vi "ejerciciofig5-Martin.vi"() -> ()   [LabVIEW 2020]
panel:
  in  "Fila":dbl[](array[numeric])
  in  "Index fila":i32
  in  "Seleccion":u8
  out "Salida":dbl[][](array[numeric])
  in  "Entrada":dbl[][](array[numeric])
  # "Digite solamente 1 o 2, segun requiera"
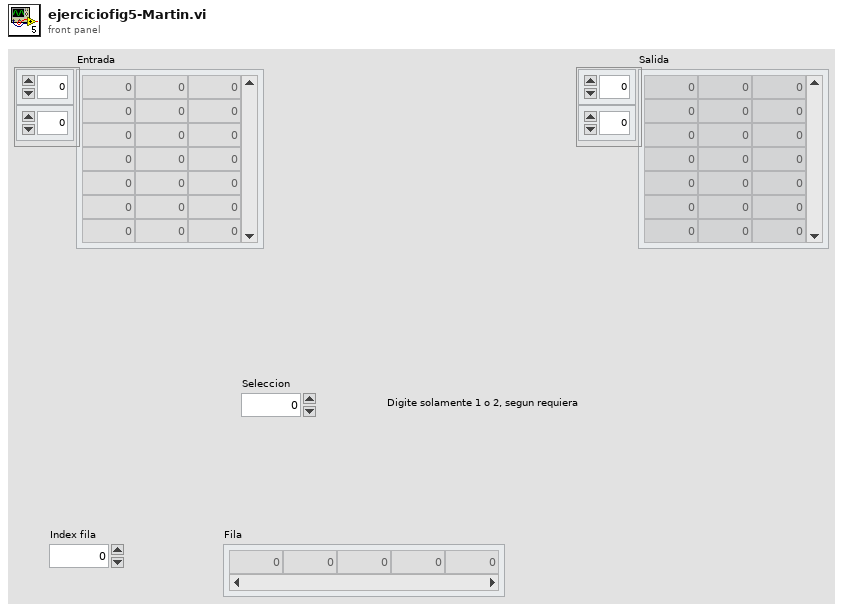
[diagram p1: front panel]
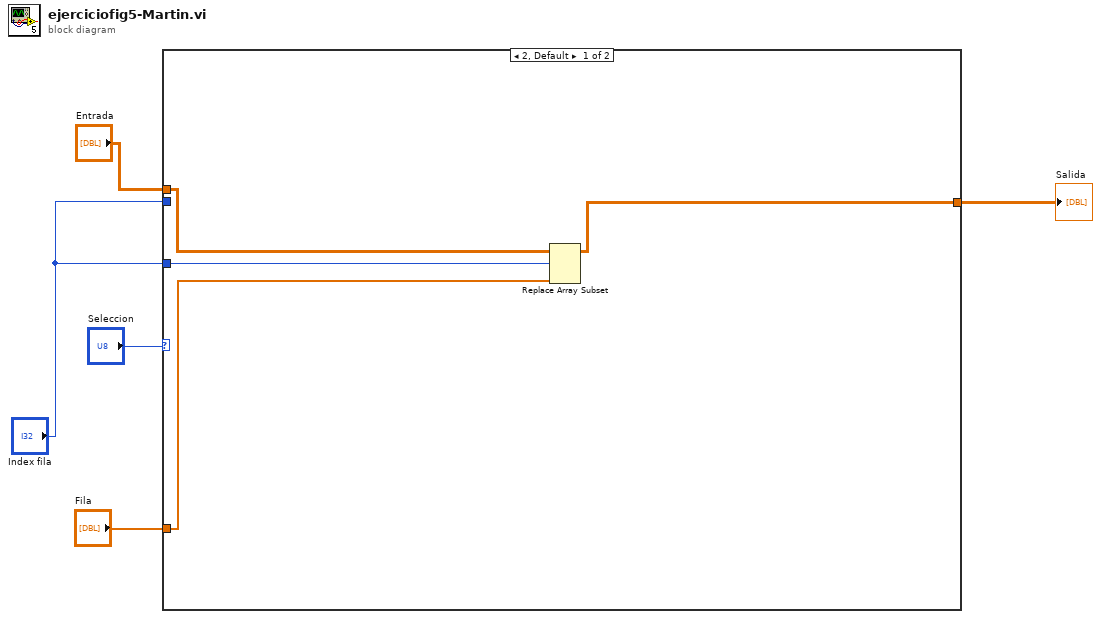
[diagram p0: block diagram]
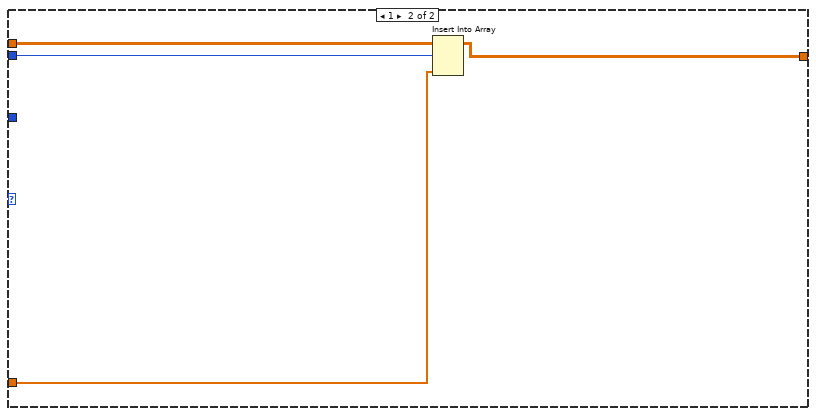
[diagram p2: hidden frame]
diagram:
  n1 = case shown="2, Default" "Seleccion" {
    tunnel: "Entrada" -> [w9 w13]
    tunnel: "Index fila" -> [_ w12]
    tunnel: "Fila" -> [w7 w11]
    tunnel: [w6 w10] -> w2
    tunnel: "Index fila" -> [w8 _]
    frame 2, Default {
      n2 = Replace Array Subset(array=w9, new element=w7, index (row)=w8) -> (w6:dbl[][])  [unwired: 1 in]
    }
    frame 1 {
      n3 = Insert Into Array(array=w13, index (row)=w12, new element=w11) -> (w10:dbl[][])  [unwired: 1 in]
    }
  }
  "Salida" <- w2
